vi "Modbus to Integer.vi"(10 "Registers In":u16[](array[numeric])) -> (2 "Values Out":u16[](array[numeric]))   [LabVIEW 2024, in "Bronkhorst Flexi-Flow ModbusTCP API.lvlib"]
uses:
  Bronkhorst Flexi-Flow ModbusTCP API.lvlib
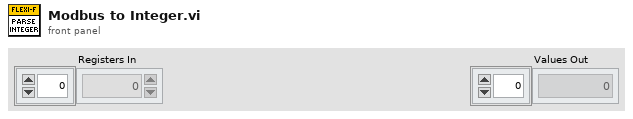
[diagram p1: front panel]
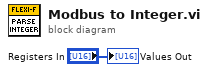
[diagram p0: block diagram]
diagram:
  "Values Out" <- "Registers In"
